vi "fgv_gps_config.vi"(7 "cmd":enum16{"read", "write"}(ring), 8 "error in":errorcluster, 11 "GNSS cfg":T1={"Port"="COM10", "rate"=115200}) -> (0 "error out":errorcluster, 3 "GNSS cfg out":T1={"Port"="COM10", "rate"=115200})   [LabVIEW 2019]
uses:
  Ctrl/gnss_config-2.ctl
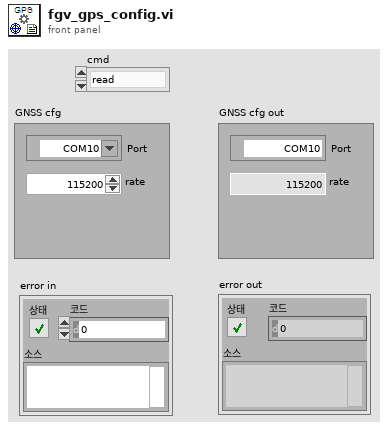
[diagram p1: front panel]
types:
  T1 = typedef "gnss_config-2.ctl" = cluster{"Port":refnum<visa-resource-name>, "rate":u32}
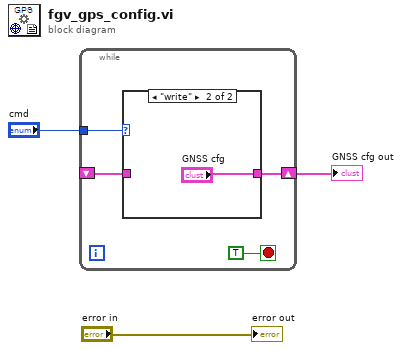
[diagram p0: block diagram]
diagram:
  n1 = while {
    tunnel: "cmd" -> [w6]
    shift-right: [w5] -> w1
    shift-left: _ -> [w4]
    stop <- TRUE stop-if-true
    n2 = case shown="\"write\"" w6 {
      tunnel: [w8 "GNSS cfg"] -> w5
      tunnel: w4 -> [w8 _]
      frame "read", Default {
      }
      frame "write" {
      }
    }
  }
  "GNSS cfg out" <- w1
  "error out" <- "error in"
